vi "Command Deliver Gear with Safety.vi"(2 "Robot System Functions In":T1, 3 "Startup":bool, 4 "String Parameter":string, 5 "Cmd Parameter 3":dbl, 6 "Cmd Parameter 2":dbl, 7 "Cmd Parameter 1":dbl) -> (0 "Robot System Functions Out":T1, 1 "Completed":bool)   [LabVIEW 2016]
uses:
  Subsystems/All Robot Commands.ctl
  Subsystems/Drive and Climb SS/Drive + Climb Commands 2017.ctl
  Subsystems/Gear Delivery SS/Gear Delivery Commands.ctl
  Subsystems/Conveyor and Shooter SS/Conveyor and Shooter Commands.ctl
  Subsystems/Ball Intake SS/Ball Intake Commands.ctl
  Command Execution State.ctl
  Global Variables/Folder Names.vi
  Global Variables/Sensor Data.vi
panel:
  in  "String Parameter 2":string
  # "Sample robot\ncontrol output.\nReplace with \nactual teleop \ncontrol signal \nstructure."
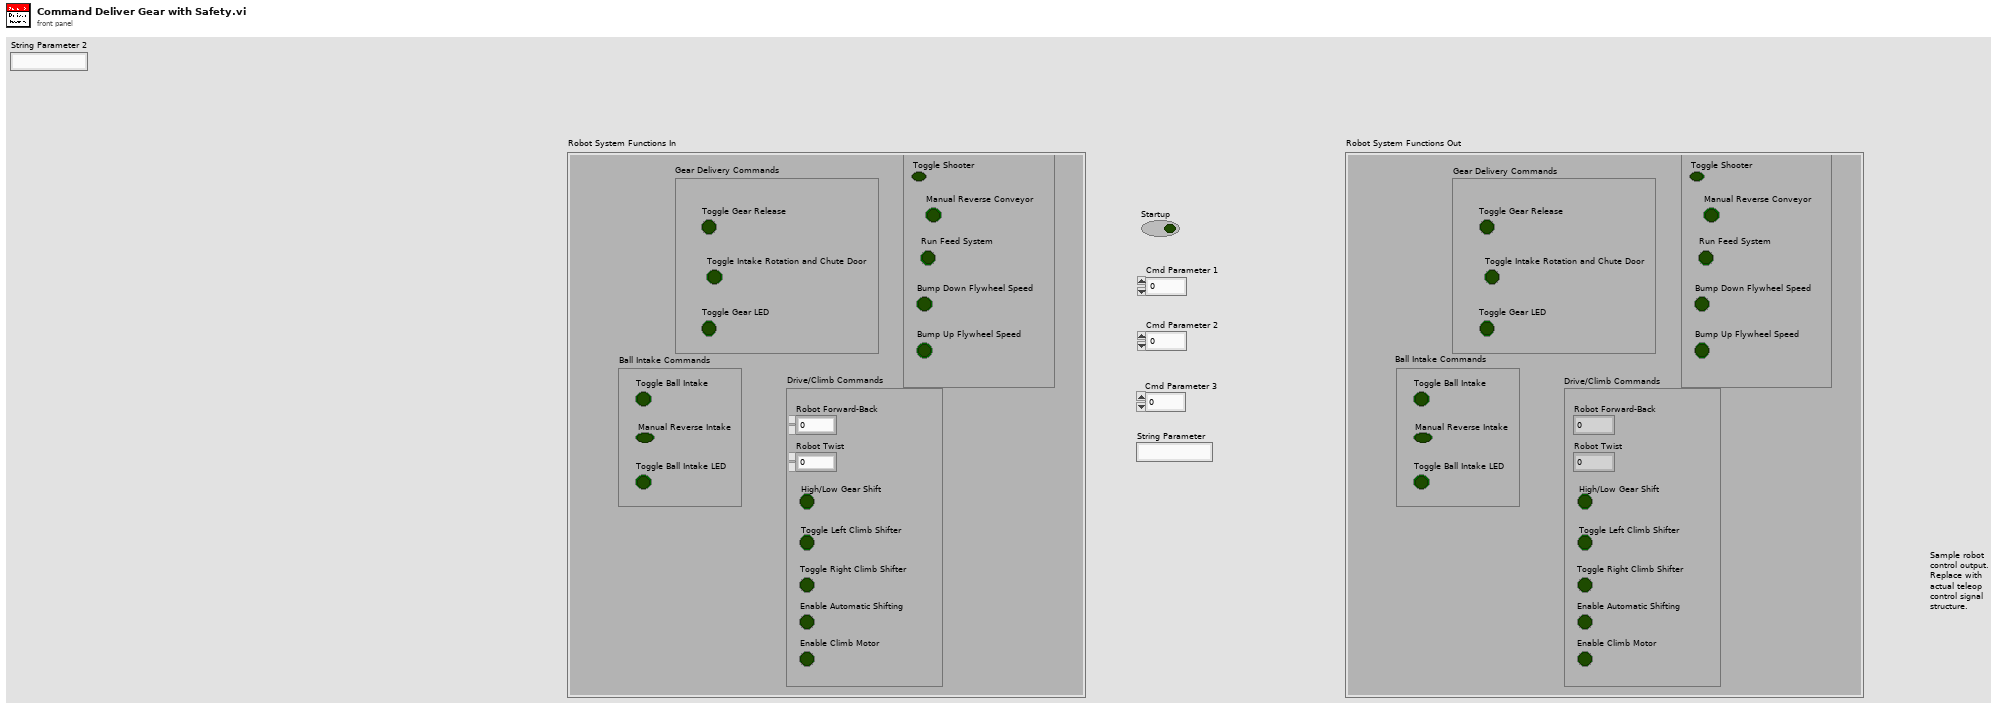
[diagram p1: front panel]
types:
  T1 = typedef "All Robot Commands.ctl" = cluster{"Drive/Climb Commands":T2, "Gear Delivery Commands":T3, "Shooter and Conveyor Commands":T4, "Ball Intake Commands":T5}
  T2 = typedef "Drive + Climb Commands 2017.ctl" = cluster{"Robot Forward-Back":dbl, "Robot Twist":dbl, "High/Low Gear Shift":bool, "Toggle Left Climb Shifter":bool, "Toggle Right Climb Shifter":bool, "Enable Automatic Shifting":bool, "Enable Climb Motor ":bool}
  T3 = typedef "Gear Delivery Commands.ctl" = cluster{"Toggle Gear Release":bool, "Toggle Intake Rotation and Chute Door":bool, "Toggle Gear LED":bool}
  T4 = typedef "Conveyor and Shooter Commands.ctl" = cluster{"Toggle Shooter":bool, "Manual Reverse Conveyor":bool, "Run Feed System":bool, "Bump Down Flywheel Speed":bool, "Bump Up Flywheel Speed":bool}
  T5 = typedef "Ball Intake Commands.ctl" = cluster{"Toggle Ball Intake":bool, "Manual Reverse Intake":bool, "Toggle Ball Intake LED":bool}
  T6 = typedef "Command Execution State.ctl" = enum16{"Initialize", "Execute", "Finish"}
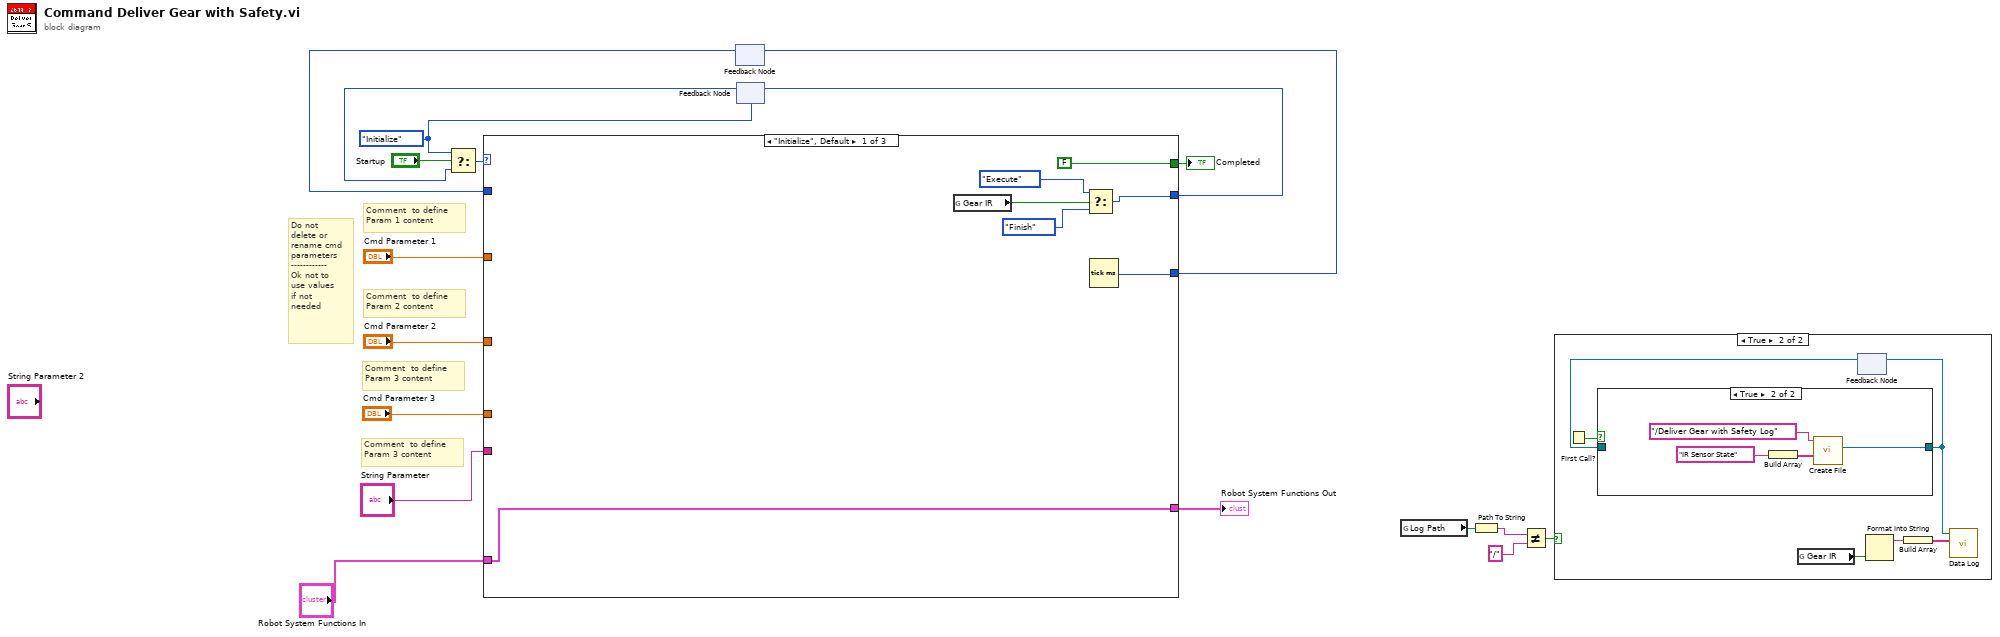
[diagram p0: block diagram]
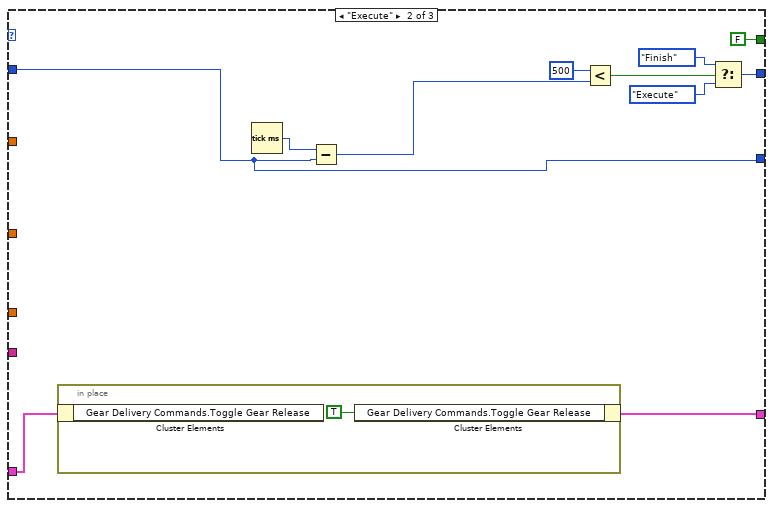
[diagram p4: hidden frame]
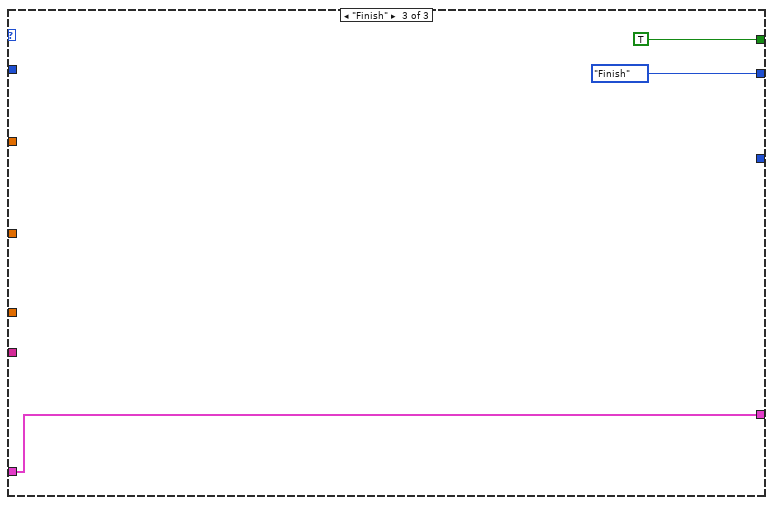
[diagram p5: hidden frame]
diagram:
  w13 = Command_Execution_State."Initialize" ("Play State")
  # "Comment  to define\nParam 3 content"
  # "Comment  to define\nParam 3 content"
  # "Do not \ndelete or\nrename cmd\nparameters\n------------\nOk not to \nuse values\nif not \nneeded"
  # "Comment  to define\nParam 2 content"
  # "Comment  to define\nParam 1 content"
  n1 = feedback #1() -> (w5:u32)  [unwired: 1 in]
  n2 = feedback #2(w13) -> (w14:T6)
  n3 = Select(t=w13, s="Startup", f=w14) -> (s? t:f=w18:T6)
  n4 = case shown="\"Initialize\", Default" w18 {
    tunnel: [FALSE FALSE TRUE] -> w16
    tunnel: [w22 w34 Command_Execution_State."Finish" ("f")] -> w15
    tunnel: "Cmd Parameter 1" -> [_ _ _]
    tunnel: "Cmd Parameter 2" -> [_ _ _]
    tunnel: [w24 w31 w38] -> w10
    tunnel: "Robot System Functions In" -> [w24 w32 w38]
    tunnel: "Cmd Parameter 3" -> [_ _ _]
    tunnel: "String Parameter" -> [_ _ _]
    tunnel: w5 -> [_ w28 _]
    tunnel: [w23 w28 _] -> w6
    frame "Initialize", Default {
      n5 = global read "Sensor Data.vi" "Gear IR"() -> (w19:bool)
      n6 = Select(t=Command_Execution_State."Execute" ("Play State"), s=w19, f=Command_Execution_State."Finish" ("Play State")) -> (s? t:f=w22:T6)
      n7 = Tick Count (ms)() -> (millisecond timer value=w23:u32)
    }
    frame "Execute" {
      n8 = in-place {
        n9 = in-place-cluster #3(w32) -> ()  [unwired: 1 out]
        n10 = in-place-cluster #3("Gear Delivery Commands.Toggle Gear Release"=TRUE ("Gear Delivery Commands.Toggle Gear Doors")) -> (w31:T1)
      }
      n11 = Tick Count (ms)() -> (millisecond timer value=w30:u32)
      n12 = Subtract(x=w30, y=w28) -> (x-y=w27:u32)
      n13 = Less?(x=u32 500, y=w27) -> (x < y?=w29:bool)
      n14 = Select(t=Command_Execution_State."Finish" ("Play State"), s=w29, f=Command_Execution_State."Execute") -> (s? t:f=w34:T6)
    }
    frame "Finish" {
    }
  }
  "Completed" <- w16
  "Robot System Functions Out" <- w10
  n15 = feedback-in #1(w6) -> ()
  n16 = feedback-in #2(w15) -> ()
  n17 = global read "Folder Names.vi" "Log Path"() -> (w4:path)
  n18 = Path To String(path=w4) -> (string=w3:string)
  n19 = Not Equal?(x=w3, y="/") -> (x != y?=w1:bool)
  n20 = case shown="True" w1 {
    frame False {
    }
    frame True {
      n21 = First Call?() -> (First Call?: T/F=w46:bool)
      n22 = global read "Sensor Data.vi" "Gear IR"() -> (w42:bool)
      n23 = feedback #4() -> (w45:refnum<file>)  [unwired: 1 in]
      n24 = case shown="True" w46 {
        tunnel: [w47 w48] -> w44
        tunnel: w45 -> [w47 _]
        frame False {
        }
        frame True {
          n25 = Build Array("IR Sensor State") -> (w50:string[])
          n26 = call "Create File.vi"("Column Titles"=w50, "File Name"="/Deliver Gear with Safety Log" ("string")) -> ("File Reference Out"=w48:refnum<file>)  [unwired: 9 in]
        }
      }
      n27 = feedback-in #4(w44) -> ()
      n28 = Format Into String(w42) -> (resulting string=w41:string)  [unwired: 3 in, 1 out]
      n29 = Build Array(w41) -> (w43:string[])
      n30 = call "Data Log.vi"("Data In"=w43, "File Reference In"=w44) -> ()  [unwired: 9 in, 1 out]
    }
  }
